vi "file directory permissions [test].vi"() -> ()   [LabVIEW 2016]
uses:
  file permissions action.ctl
panel:
  in  "others":T1={"read"=TRUE, "write"=TRUE, "execute"=TRUE}
  in  "group":T1={"read"=TRUE, "write"=TRUE, "execute"=TRUE}
  out "error out":errorcluster
  out "directory out":path
  out "reset permissions":i16 format="%o"
  out "reset?":bool
  out "changed?":bool
  out "new permissions":i16 format="%o"
  in  "owner":T1={"read"=TRUE, "write"=TRUE, "execute"=TRUE}
  in  "file directory (default data)":path
  out "original permissions":i16 format="%o"
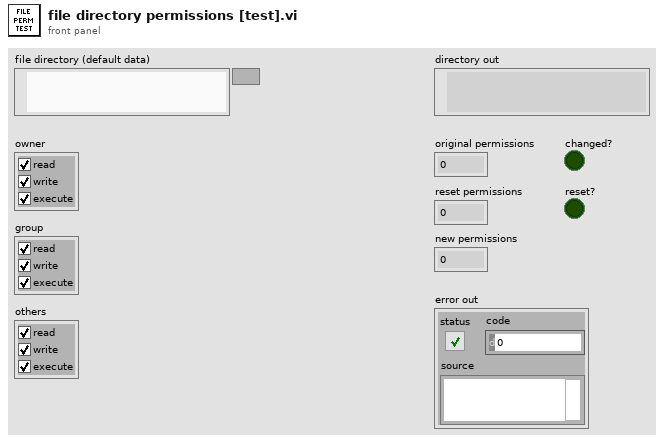
[diagram p1: front panel]
types:
  T1 = cluster{"read":bool, "write":bool, "execute":bool}
  T2 = typedef "file permissions action.ctl" = enum16{"get", "set", "reset"}
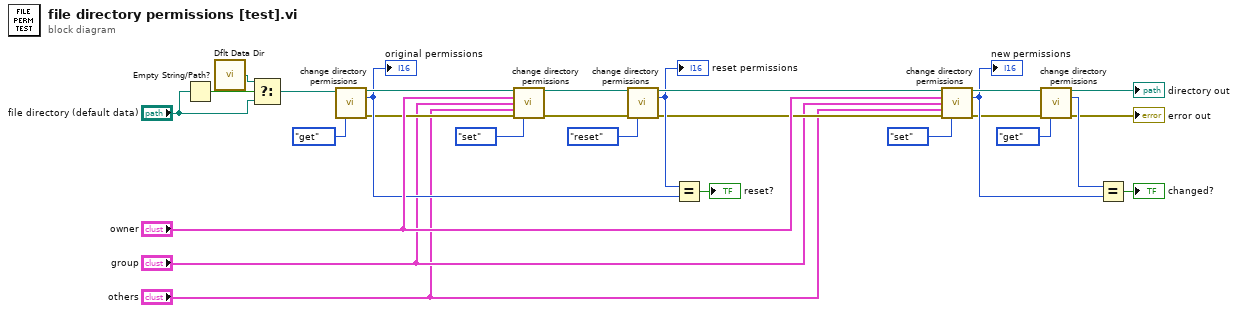
[diagram p0: block diagram]
diagram:
  n1 = Empty String/Path?(string/path="file directory (default data)") -> (empty?=w12:bool)
  n2 = call <vilib>:"Dflt Data Dir.vi"() -> ("App:Default Data Directory"=w11:path)
  n3 = Select(t=w11, s=w12, f="file directory (default data)") -> (s? t:f=w9:path)
  n4 = call "change directory permissions.vi"("directory"=w9, "action (get)"=file_permissions_action."get") -> ("directory out"=w21:path, "permissions"=w14:i16, "error out"=w7:errorcluster)  [unwired: 11 in]
  "original permissions" <- w14
  n5 = call "change directory permissions.vi"("directory"=w21, "owner"="owner", "group"="group", "others"="others", "error in"=w7, "action (get)"=file_permissions_action."set") -> ("directory out"=w20:path, "error out"=w6:errorcluster)  [unwired: 7 in, 1 out]
  n6 = call "change directory permissions.vi"("directory"=w20, "error in"=w6, "action (get)"=file_permissions_action."reset") -> ("directory out"=w19:path, "permissions"=w15:i16, "error out"=w5:errorcluster)  [unwired: 10 in]
  "reset permissions" <- w15
  n7 = Equal?(x=w15, y=w14) -> (x = y?=→"reset?":bool)
  n8 = call "change directory permissions.vi"("directory"=w19, "owner"="owner", "group"="group", "others"="others", "error in"=w5, "action (get)"=file_permissions_action."set") -> ("directory out"=w18:path, "permissions"=w13:i16, "error out"=w4:errorcluster)  [unwired: 7 in]
  "new permissions" <- w13
  n9 = call "change directory permissions.vi"("directory"=w18, "error in"=w4, "action (get)"=file_permissions_action."get") -> ("directory out"=→"directory out":path, "permissions"=w16:i16, "error out"=→"error out":errorcluster)  [unwired: 10 in]
  n10 = Equal?(x=w16, y=w13) -> (x = y?=→"changed?":bool)
